vi "Alarm Log RT.vi"(8 "error in (no error)":errorcluster, 11 "Network Path":string="172.22.26.202") -> (2 "AlarmLog out":string[][](array[string]), 3 "Network Path":string="172.22.26.202")   [LabVIEW 2018]
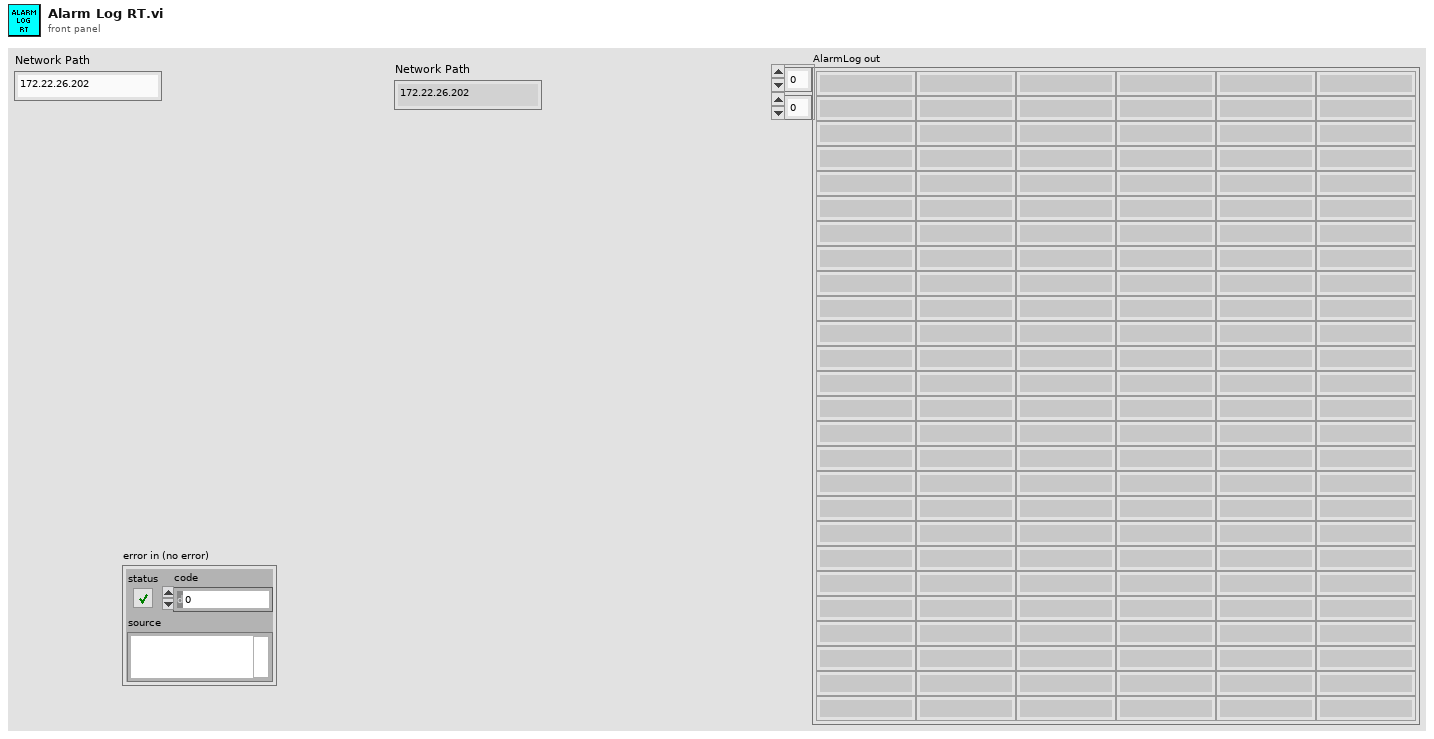
[diagram p1: front panel]
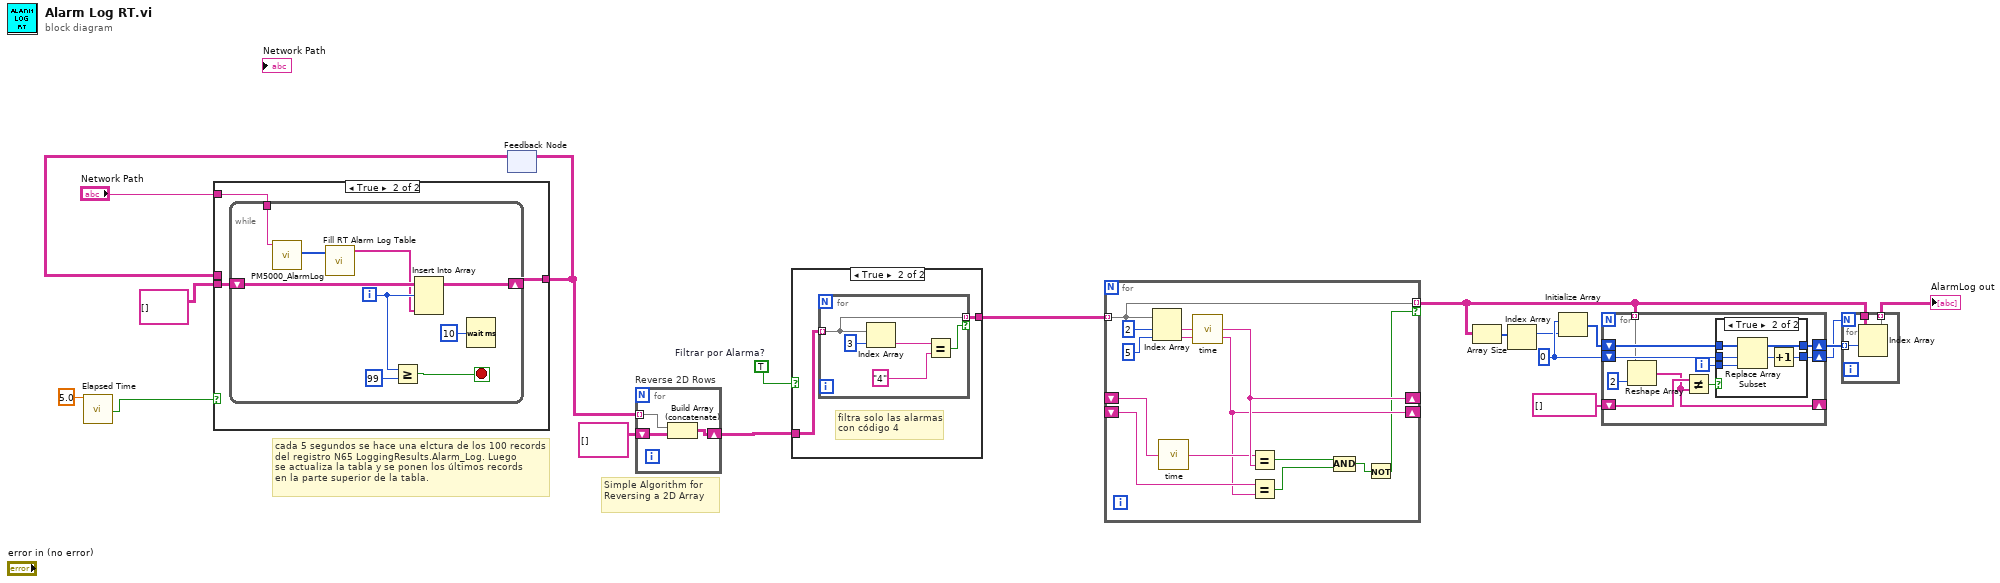
[diagram p0: block diagram]
diagram:
  w7 = 0
  w14 = TRUE  # Filtrar por Alarma?
  # "Simple Algorithm for Reversing a 2D Array"
  # "cada 5 segundos se hace una elctura de los 100 records\ndel registro N65 LoggingResults.Alarm_Log. Luego\nse actualiza la tabla y se ponen los últimos records \nen la parte superior de la tabla."
  n1 = call "Elapsed Time"("Time Target (s)"=5.0) -> ("Time has Elapsed"=w17:bool)  [unwired: 11 in, 7 out]
  n2 = feedback #1() -> (w12:string[][])  [unwired: 1 in]
  n3 = case shown="True" w17 {
    tunnel: string[][] [] -> [_ w23]
    tunnel: [w20 w22] -> w13
    tunnel: w12 -> [w20 _]
    tunnel: "Network Path" -> [_ w21]
    frame False {
    }
    frame True {
      n4 = while {
        shift-right: [w31] -> w22
        shift-left: w23 -> [w32]
        tunnel: w21 -> [w25]
        i -> [w30]
        stop <- w28 stop-if-true
        n5 = call "PM5000_AlarmLog.vi"("Network Path"=w25) -> ("Alarm Log"=w24:i16[])  [unwired: 8 in, 2 out]
        n6 = call "Fill RT Alarm Log Table.vi"("Alarm Log"=w24) -> ("appended array"=w26:string[])  [unwired: 10 in]
        n7 = Greater Or Equal?(x=w30, y=99) -> (x >= y?=w28:bool)
        n8 = Insert Into Array(array=w32, index (row)=w30, new element=w26) -> (w31:string[][])  [unwired: 1 in]
        n9 = Wait (ms)(milliseconds to wait=u32 10) -> ()  [unwired: 1 out]
      }
    }
  }
  n10 = feedback-in #1(w13) -> ()
  n11 = for "Reverse 2D Rows" {
    tunnel: w13 -> [w35] mode=indexing
    shift-right: [w33] -> w15
    shift-left: string[][] [] -> [w34]
    n12 = Build Array (concatenate)(w35, w34) -> (w33:string[][])
  }
  n13 = case shown="True" w14 {
    tunnel: w15 -> [w36 w38]
    tunnel: [w36 w37] -> w10
    frame False {
    }
    frame True {
      # "filtra solo las alarmas\ncon código 4"
      n14 = for {
        tunnel: w38 -> [w43] mode=indexing
        tunnel: [w43] -> w37 mode=indexing if=w39
        n15 = Index Array(array=w43, index=3) -> (element=w41:string)
        n16 = Equal?(x=w41, y="4" ("Filtro")) -> (x = y?=w39:bool)
      }
    }
  }
  n17 = for {
    tunnel: w10 -> [w56] mode=indexing
    tunnel: [w56] -> w2 mode=indexing if=w44
    shift-right: [w47] -> _
    shift-left: _ -> [w50]
    shift-right: [w45] -> _
    shift-left: _ -> [w52]
    n18 = Index Array(array=w56, index #1=2 ("index"), index #2=5 ("index")) -> (element #1=w48:string, element #2=w45:string)
    n19 = call "time.vi"("in"=w50) -> ("out"=w46:string)
    n20 = call "time.vi"("in"=w48) -> ("out"=w47:string)
    n21 = Equal?(x=w46, y=w47) -> (x = y?=w54:bool)
    n22 = Equal?(x=w52, y=w45) -> (x = y?=w51:bool)
    n23 = Compound Arithmetic op=AND(w54, w51) -> (w49:bool)
    n24 = Not(x=w49) -> (.not. x?=w44:bool)
  }
  n25 = Array Size(array=w2) -> (size(s)=w9:i32[])
  n26 = Index Array(array=w9) -> (element=w3:i32)  [unwired: 1 in]
  n27 = Initialize Array(w7, w3) -> (w8:i32[])
  n28 = for {
    shift-right: [w57] -> _
    shift-left: string[] [] ("Sample Data") -> [w58]
    shift-right: [w65] -> w6
    shift-left: w8 -> [w66]
    shift-right: [w63] -> w4
    shift-left: w7 -> [w64]
    tunnel: w2 -> [w60] mode=indexing
    i -> [w61]
    n29 = Reshape Array(w60, 2 ("dimension size")) -> (w57:string[])
    n30 = Not Equal?(x=w58, y=w57) -> (x != y?=w62:bool)
    n31 = case shown="True" w62 {
      tunnel: w66 -> [w67 w73]
      tunnel: [w67 w72] -> w65
      tunnel: w64 -> [w68 w71]
      tunnel: [w68 w70] -> w63
      tunnel: w61 -> [_ w69]
      frame False {
      }
      frame True {
        n32 = Replace Array Subset(array=w73, new element=w69, index=w71) -> (w72:i32[])
        n33 = Increment(x=w71) -> (x+1=w70:i32)
      }
    }
  }
  n34 = for {
    N: w4 -> [_]
    tunnel: w2 -> [w76]
    tunnel: w6 -> [w75] mode=indexing
    tunnel: [w74] -> w1 mode=indexing
    n35 = Index Array(array=w76, index (row)=w75) -> (element=w74:string[])  [unwired: 1 in]
  }
  "AlarmLog out" <- w1
